vi "Get Default.vi"(8 "error in (no error)":errorcluster, 11 "Tree in":refnum<class "Tree.lvclass">) -> (0 "error out":errorcluster, 2 "Node out":refnum<class "TreeNode.lvclass">, 3 "Tree out":refnum<class "Tree.lvclass">)   [LabVIEW 2013, in "MDSplus.lvlib" / "Tree.lvclass"]
doc: "Get the TreeNode for the default node."
uses:
  <vilib>/MDSplus/Classes/Tree_Class/Tree.lvclass
  <vilib>/MDSplus/Classes/Data_Class/TreeNode_Class/TreeNode.lvclass
  <vilib>/MDSplus/Classes/Data_Class/Data.lvclass
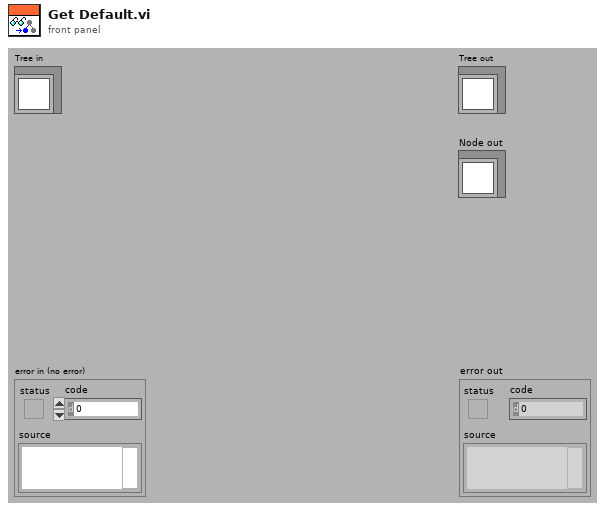
[diagram p1: front panel]
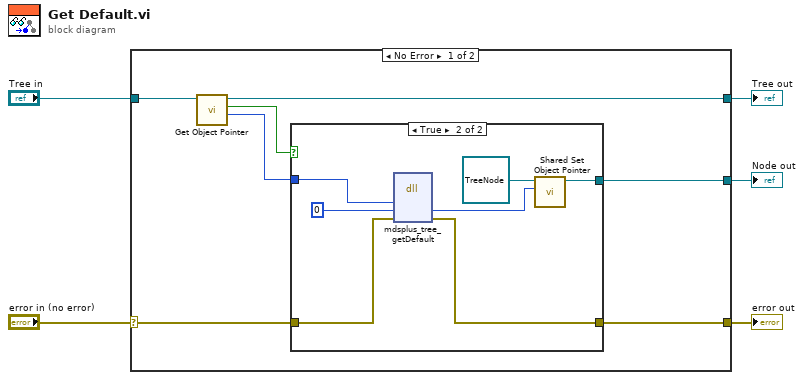
[diagram p0: block diagram]
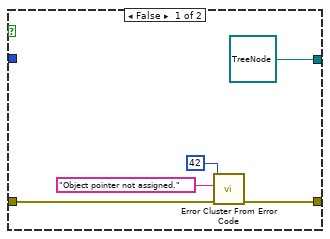
[diagram p2: hidden frame]
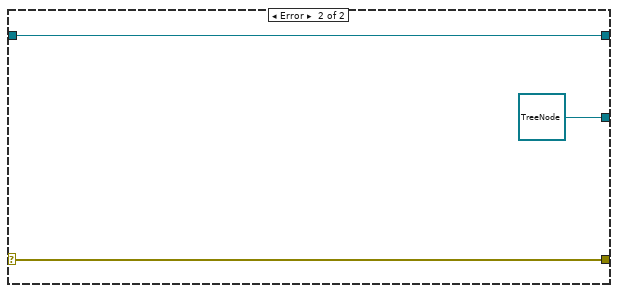
[diagram p3: hidden frame]
diagram:
  n1 = case shown="No Error" "error in (no error)" {
    selector: "error in (no error)" -> [w7 w27]
    tunnel: [w6 w27] -> w4
    tunnel: [w11 w26] -> w2
    tunnel: "Tree in" -> [w12 w26]
    tunnel: [w10 refnum<class "TreeNode.lvclass"> refnum ("TreeNode out")] -> w1
    frame No Error {
      n2 = call-dynamic "Get Object Pointer.vi"("Tree in"=w12) -> ("Object Pointer"=w8:i64, "Assigned object pointer?"=w9:bool, "Tree out"=w11:refnum<class "Tree.lvclass">)  [unwired: 8 in]
      n3 = case shown="True" w9 {
        tunnel: [refnum<class "TreeNode.lvclass"> refnum ("Data out") w21] -> w10
        tunnel: w8 -> [_ w20]
        tunnel: w7 -> [w14 w19]
        tunnel: [w13 w18] -> w6
        frame False {
          n4 = call <vilib>:"Error Cluster From Error Code.vi"("error in (no error)"=w14, "error message (\"\")"="Object pointer not assigned." ("error message (\"\")"), "error code (0)"=42) -> ("error out"=w13:errorcluster)  [unwired: 6 in]
        }
        frame True {
          n5 = dll-call lib="MDSobjectsLVShr" fn="mdsplus_tree_getDefault"("lvTreePtr"=w20, "lvTreeNodePtrOut"=i64 0 ("lvTreeNodePtr"), "error"=w19) -> ("lvTreeNodePtrOut"=w22:i64, "error"=w18:errorcluster)  [unwired: 5 in, 2 out]
          n6 = call <vilib>:"Shared Set Object Pointer.vi"("Object Pointer"=w22, "Data in"=refnum<class "TreeNode.lvclass"> refnum ("TreeNode")) -> ("Data out"=w21:refnum<class "TreeNode.lvclass">)  [unwired: 9 in]
        }
      }
    }
    frame Error {
    }
  }
  "error out" <- w4
  "Tree out" <- w2
  "Node out" <- w1
